vi "LC-MISDK_SetMeasurementCondition.vi"() -> ()   [LabVIEW 2015]
uses:
  C:/Users/e09031/Documents/GMA/LC-160/Labview/Sample_LC-MISDK/LC-MISDK.dll
  LC-MISDK.dll
panel:
  in  "SetCalibCh":bool
  out "GetCalibCh":dbl
  out "CalibError":dbl
  in  "SetCalibCh":dbl
  out "SyncError":dbl
  out "Error":dbl
  out "PeakValley":string
  out "SyncMode":string
  out "Frequency":dbl
  out "MeasTimeMode":string
  out "ManualMeasTime":dbl
  out "GetLight":bool
  in  "キャンセルボタン":bool
  in  "SetPeakValley":enum32{"OFF", "Peak", "Valley"}(radio)
  in  "SetSync":bool
  in  "Frequency":dbl[unit]
  in  "SetTime":bool
  in  "MeasurementTime":dbl[unit] format="%#_6f"
  out "BackLibhtLED":bool
  in  "BackLight":bool
  # "SetSyncMode"
  # "SetBackLight"
  # "GetBackLight"
  # "GetSyncMode"
  # "Hz"
  # "SetMeasurementTime"
  # "SetCalibrationCh"
  # "GetMeasurementTime"
  # "GetCalibrationCh"
  # "GetPeakValley"
  # "S"
  # "Auto"
  # "Manual"
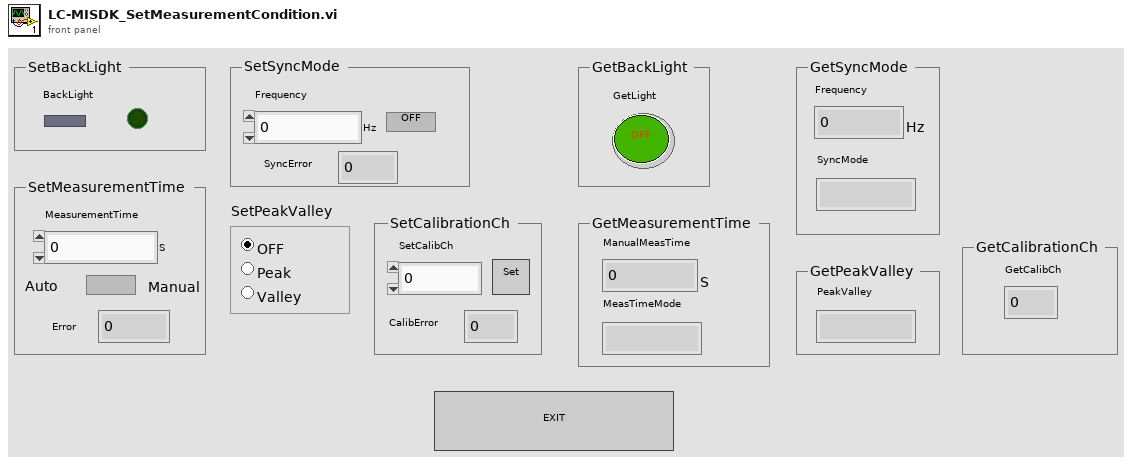
[diagram p1: front panel]
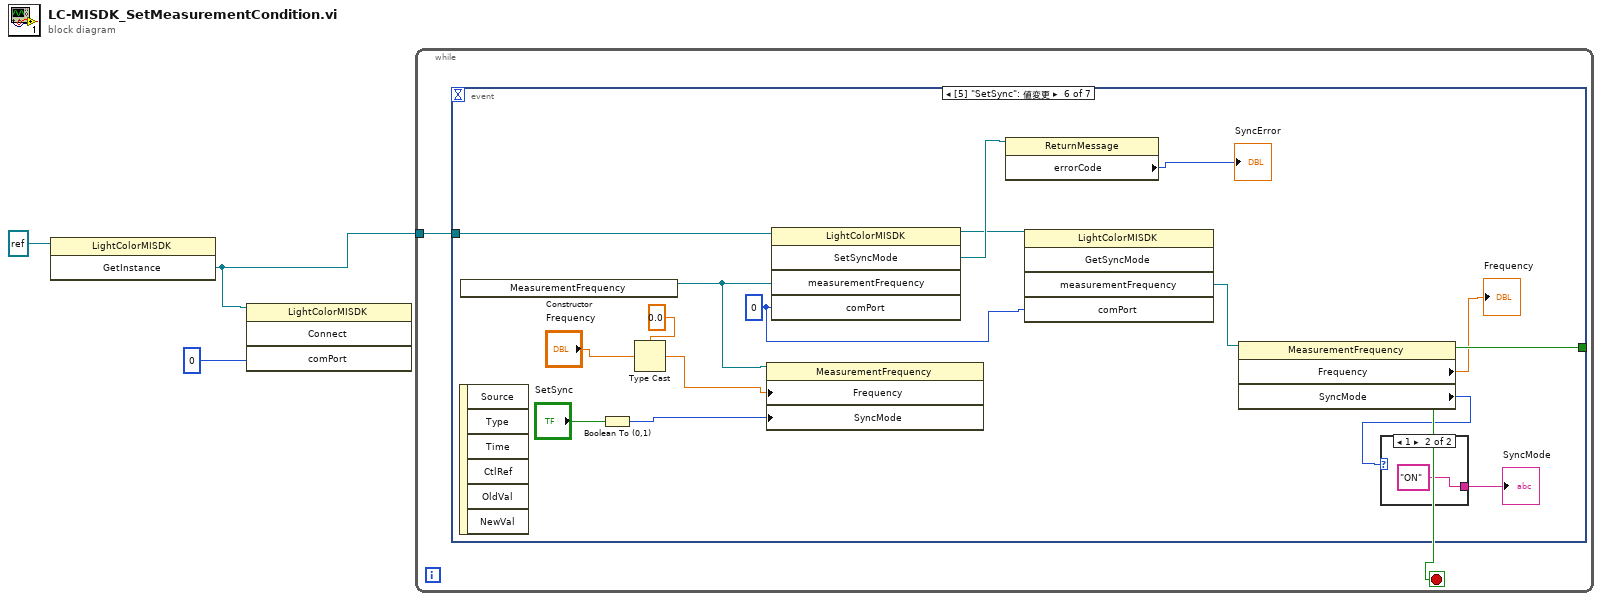
[diagram p0: block diagram]
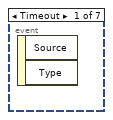
[diagram p2: hidden frame]
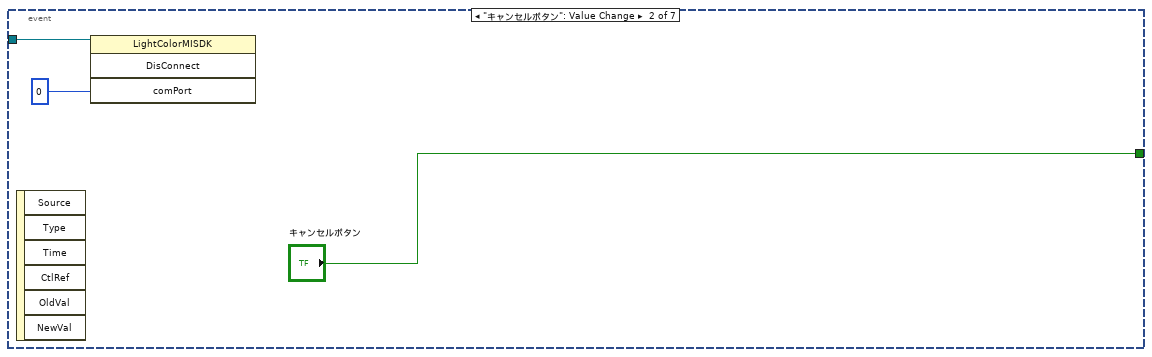
[diagram p3: hidden frame]
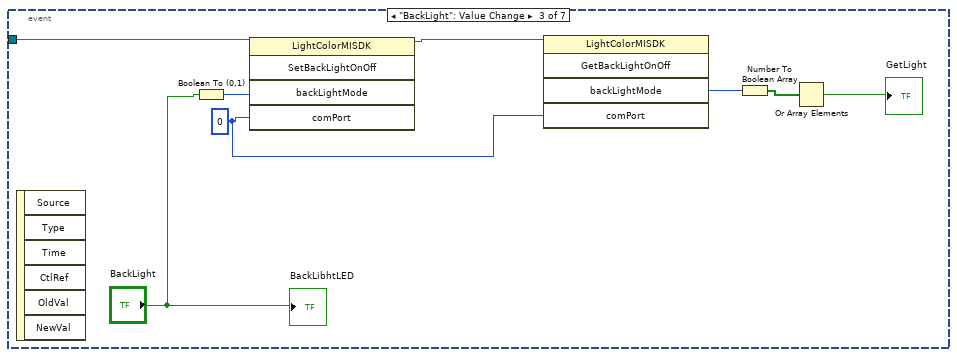
[diagram p4: hidden frame]
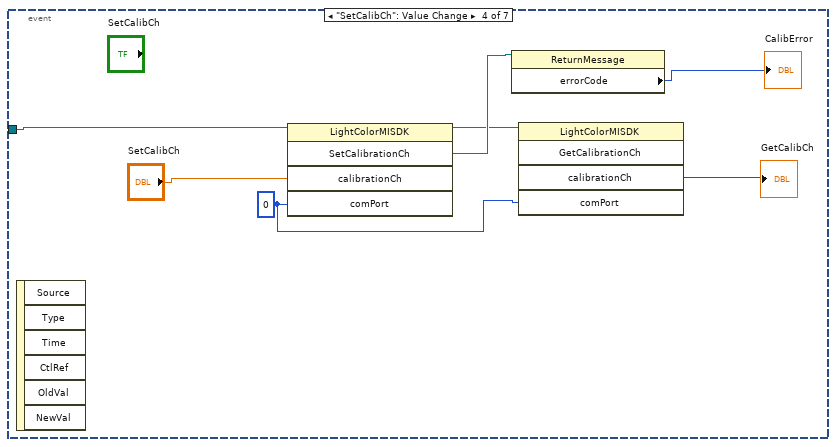
[diagram p5: hidden frame]
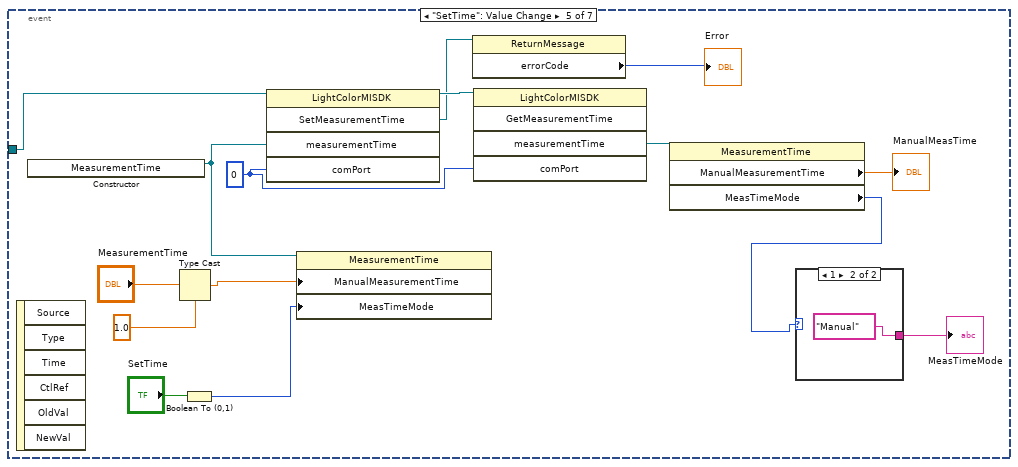
[diagram p6: hidden frame]
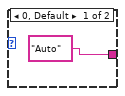
[diagram p7: hidden frame]
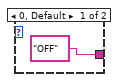
[diagram p8: hidden frame]
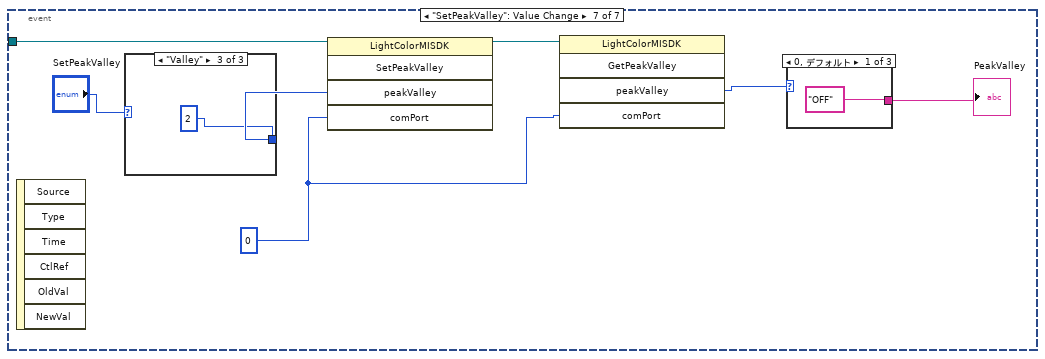
[diagram p9: hidden frame]
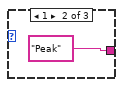
[diagram p10: hidden frame]
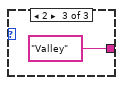
[diagram p11: hidden frame]
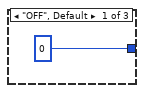
[diagram p12: hidden frame]
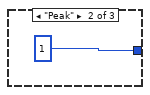
[diagram p13: hidden frame]
diagram:
  n1 = invoke on="インボークノード" class="LightColorMISDK" method="GetInstance"(reference=refnum<k24> refnum ("リファレンス出力")) -> ("GetInstance"=w2:refnum<k24>)  [unwired: 2 in, 2 out]
  n2 = invoke on="インボークノード" class="LightColorMISDK" method="Connect"(reference=w2, "comPort"=0) -> ()  [unwired: 2 in, 4 out]
  n3 = while {
    tunnel: w2 -> [w4]
    stop <- w5 stop-if-true
    n4 = event shown="[5] \"SetSync\": 値変更" {
      selector: _ -> [_ _ _ _ _ _ _]
      dyn-events: _ -> [_ _ _ _ _ _ _]
      timeout: _ -> [_ _ _ _ _ _ _]
      tunnel: [_ "キャンセルボタン" _ _ _ _ _] -> w5
      tunnel: w4 -> [_ w6 w16 w23 w38 w55 w62]
      event Timeout {
        n5 = event-data() -> ()  [unwired: 1 in, 2 out]
      }
      event "キャンセルボタン": Value Change {
        n6 = event-data() -> ()  [unwired: 1 in, 6 out]
        n7 = invoke on="インボークノード" class="LightColorMISDK" method="DisConnect"(reference=w6, "comPort"=0) -> ()  [unwired: 2 in, 4 out]
      }
      event "BackLight": Value Change {
        w12 = 0
        n8 = event-data() -> ()  [unwired: 1 in, 6 out]
        n9 = Boolean To (0,1)(Boolean="BackLight") -> (0, 1=w14:i16)
        n10 = invoke on="インボークノード" class="LightColorMISDK" method="SetBackLightOnOff"(reference=w16, "backLightMode"=w14, "comPort"=w12) -> (reference out=w13:refnum<k24>)  [unwired: 2 in, 4 out]
        n11 = invoke on="インボークノード" class="LightColorMISDK" method="GetBackLightOnOff"(reference=w13, "comPort"=w12) -> ("backLightMode"=w11:i32)  [unwired: 3 in, 4 out]
        n12 = Number To Boolean Array(number=w11) -> (Boolean array=w10:bool[])
        n13 = Or Array Elements(Boolean array=w10) -> (logical OR=→"GetLight":bool)
        "BackLibhtLED" <- "BackLight"
      }
      event "SetCalibCh": Value Change {
        w18 = 0
        n14 = event-data() -> ()  [unwired: 1 in, 6 out]
        n15 = invoke on="インボークノード" class="LightColorMISDK" method="SetCalibrationCh"(reference=w23, "calibrationCh"="SetCalibCh", "comPort"=w18) -> (reference out=w19:refnum<k24>, "SetCalibrationCh"=w20:refnum<k24>)  [unwired: 2 in, 3 out]
        n16 = property on="プロパティノード" class="ReturnMessage"(reference=w20) -> ("errorCode"=→"CalibError":i32)  [unwired: 1 in, 2 out]
        n17 = invoke on="インボークノード" class="LightColorMISDK" method="GetCalibrationCh"(reference=w19, "comPort"=w18) -> ("calibrationCh"=→"GetCalibCh":i32)  [unwired: 3 in, 4 out]
      }
      event "SetTime": Value Change {
        w30 = 0
        n18 = event-data() -> ()  [unwired: 1 in, 6 out]
        n19 = constructor class="MeasurementTime"() -> (reference out=w36:refnum<k24>)  [unwired: 3 in, 2 out]
        n20 = Type Cast(type=1.0, x="MeasurementTime") -> (*(type *) &x=w33:dbl)
        n21 = Boolean To (0,1)(Boolean="SetTime") -> (0, 1=w35:i16)
        n22 = invoke on="インボークノード" class="LightColorMISDK" method="SetMeasurementTime"(reference=w38, "measurementTime"=w36, "comPort"=w30) -> (reference out=w31:refnum<k24>, "SetMeasurementTime"=w25:refnum<k24>)  [unwired: 2 in, 3 out]
        n23 = property class="MeasurementTime"(reference=w36, "ManualMeasurementTime"=w33, "MeasTimeMode"=w35) -> ()  [unwired: 1 in, 2 out]
        n24 = property on="プロパティノード" class="ReturnMessage"(reference=w25) -> ("errorCode"=→"Error":i32)  [unwired: 1 in, 2 out]
        n25 = invoke on="インボークノード" class="LightColorMISDK" method="GetMeasurementTime"(reference=w31, "comPort"=w30) -> ("measurementTime"=w29:refnum<k24>)  [unwired: 3 in, 4 out]
        n26 = property on="プロパティノード" class="MeasurementTime"(reference=w29) -> ("ManualMeasurementTime"=→"ManualMeasTime":dbl, "MeasTimeMode"=w27:i32)  [unwired: 1 in, 2 out]
        n27 = case shown="1" w27 {
          tunnel: ["Auto" "Manual"] -> w26
          frame 0, Default {
          }
          frame 1 {
          }
        }
        "MeasTimeMode" <- w26
      }
      event "SetSync": Value Change {
        w45 = 0
        n28 = event-data() -> ()  [unwired: 1 in, 6 out]
        n29 = constructor class="MeasurementFrequency"() -> (reference out=w52:refnum<k24>)  [unwired: 3 in, 2 out]
        n30 = Boolean To (0,1)(Boolean="SetSync") -> (0, 1=w53:i16)
        n31 = Type Cast(type=0.0, x="Frequency") -> (*(type *) &x=w49:dbl)
        n32 = property class="MeasurementFrequency"(reference=w52, "Frequency"=w49, "SyncMode"=w53) -> ()  [unwired: 1 in, 2 out]
        n33 = invoke on="インボークノード" class="LightColorMISDK" method="SetSyncMode"(reference=w55, "measurementFrequency"=w52, "comPort"=w45) -> (reference out=w46:refnum<k24>, "SetSyncMode"=w47:refnum<k24>)  [unwired: 2 in, 3 out]
        n34 = property on="プロパティノード" class="ReturnMessage"(reference=w47) -> ("errorCode"=→"SyncError":i32)  [unwired: 1 in, 2 out]
        n35 = invoke on="インボークノード" class="LightColorMISDK" method="GetSyncMode"(reference=w46, "comPort"=w45) -> ("measurementFrequency"=w41:refnum<k24>)  [unwired: 3 in, 4 out]
        n36 = property on="プロパティノード" class="MeasurementFrequency"(reference=w41) -> ("Frequency"=→"Frequency":dbl, "SyncMode"=w43:i32)  [unwired: 1 in, 2 out]
        n37 = case shown="1" w43 {
          tunnel: ["OFF" "ON"] -> w42
          frame 0, Default {
          }
          frame 1 {
          }
        }
        "SyncMode" <- w42
      }
      event "SetPeakValley": Value Change {
        w60 = 0
        n38 = event-data() -> ()  [unwired: 1 in, 6 out]
        n39 = case shown="\"Valley\"" "SetPeakValley" {
          tunnel: [0 1 2] -> w63
          frame "OFF", Default {
          }
          frame "Peak" {
          }
          frame "Valley" {
          }
        }
        n40 = invoke on="インボークノード" class="LightColorMISDK" method="SetPeakValley"(reference=w62, "peakValley"=w63, "comPort"=w60) -> (reference out=w61:refnum<k24>)  [unwired: 2 in, 4 out]
        n41 = invoke on="インボークノード" class="LightColorMISDK" method="GetPeakValley"(reference=w61, "comPort"=w60) -> ("peakValley"=w59:i32)  [unwired: 3 in, 4 out]
        n42 = case shown="0, デフォルト" w59 {
          tunnel: ["OFF" "Peak" "Valley"] -> w58
          frame 0, Default {
          }
          frame 1 {
          }
          frame 2 {
          }
        }
        "PeakValley" <- w58
      }
    }
  }
